vi "MCP23S17 Read LATCH.vi"(8 "error in (no error)":errorcluster, 10 "Addr":T1 items=["Addr-0"=0, "Addr-1"=4, "Addr-2"=2, "Addr-3"=6, "Addr-4"=1, "Addr-5"=5, "Addr-6"=3, "Addr-7"=7], 11 "handle":u32 format="%08x") -> (0 "error out":errorcluster, 2 "LATCH":u16, 3 "handle out":u32, 5 "buffer out B":string, 7 "buffer out A":string)   [LabVIEW 2018]
uses:
  PROJEKT/NIKO/Labview/Niko V4/FTDI SPI/Ctl/Sub Addr.ctl
  PROJEKT/NIKO/Labview/Niko V5/FTDI SPI/libMPSSE-SPI.lvlib
panel:
  out "string":string
  in  "Array U8":u8[](array[numeric])=[64, 18, 0, 128, 0, 0, 0, 0, 0, 0] format="%x"
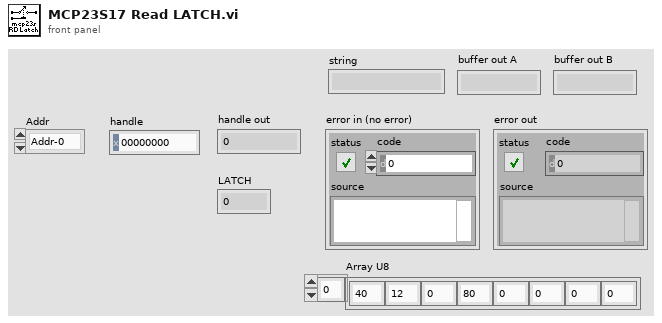
[diagram p1: front panel]
types:
  T1 = typedef "Sub Addr.ctl" = u16
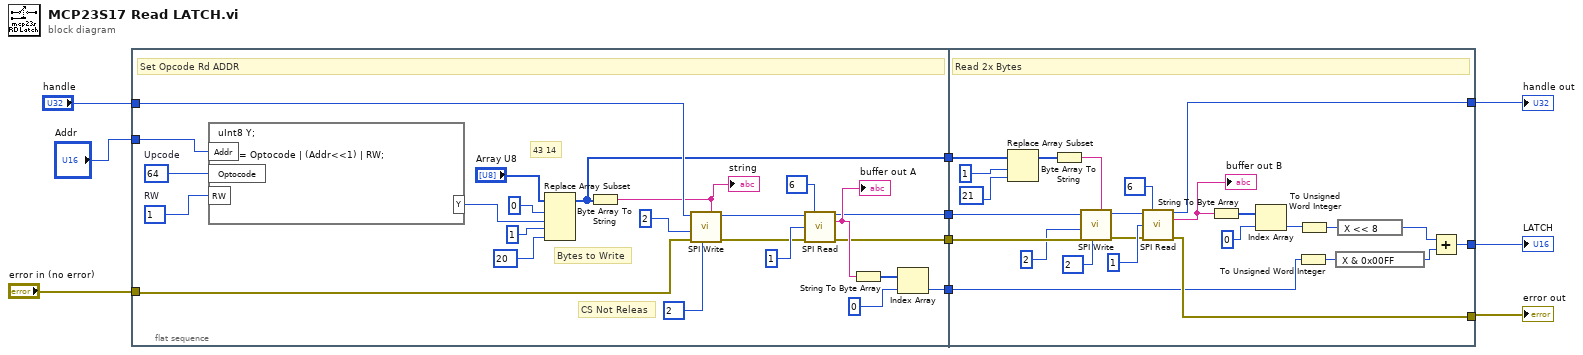
[diagram p0: block diagram]
diagram:
  n1 = flat-sequence {
    tunnel: "Addr" -> [w33]
    tunnel: "handle" -> [w29]
    tunnel: "error in (no error)" -> [w26]
    tunnel: [w14] -> w6
    tunnel: [w13] -> w5
    tunnel: [w12] -> w4
    tunnel: [w11] -> w3
    tunnel: [w57] -> w8
    tunnel: [w56] -> w2
    tunnel: [w51] -> w7
    tunnel: w6 -> [w50]
    tunnel: w5 -> [w46]
    tunnel: w4 -> [w44]
    tunnel: w3 -> [w35]
    frame #0 {
      w22 = u8 64  # Upcode
      w23 = u8 1  # RW
      # "CS Not Releas"
      # "Bytes to Write"
      # "43 14"
      # "Set Opcode Rd ADDR"
      n2 = formula code="uInt8 Y;\n      \n    Y = Optocode | (Addr<<1) | RW;"("Addr"=w33, "Optocode"=w22, "RW"=w23) -> ("Y"=w32:u8)
      n3 = Replace Array Subset(array="Array U8", new element #1=w32, index #1=0 ("index"), new element #2=u8 20, index #2=u8 1 ("new element/subarray")) -> (w14:u8[])
      n4 = Byte Array To String(unsigned byte array=w14) -> (string=w28:string)
      "string" <- w28
      n5 = call "SPI Write.vi"("buffer"=w28, "options"=u8 2, "error in (no error)"=w26, "Bytes To Send"=u32 2, "handle"=w29) -> ("error out"=w18:errorcluster, "handle out"=w19:u32)  [unwired: 4 in, 1 out]
      n6 = call "SPI Read.vi"("handle"=w19, "options"=u8 6, "sizeToTransfer"=u32 1, "error in (no error)"=w18) -> ("handle out"=w13:u32, "buffer out"=w15:string, "error out"=w12:errorcluster)  [unwired: 7 in, 2 out]
      "buffer out A" <- w15
      n7 = String To Byte Array(string=w15) -> (unsigned byte array=w16:u8[])
      n8 = Index Array(array=w16, index=0) -> (element=w11:u8)
    }
    frame #1 {
      # "Read 2x Bytes"
      n9 = Replace Array Subset(array=w50, new element=u8 21, index=u8 1 ("new element/subarray")) -> (w47:u8[])
      n10 = Byte Array To String(unsigned byte array=w47) -> (string=w45:string)
      n11 = call "SPI Write.vi"("buffer"=w45, "options"=u8 2, "error in (no error)"=w44, "Bytes To Send"=u32 2, "handle"=w46) -> ("error out"=w43:errorcluster, "handle out"=w42:u32)  [unwired: 4 in, 1 out]
      n12 = call "SPI Read.vi"("handle"=w42, "options"=u8 6, "sizeToTransfer"=u32 1, "error in (no error)"=w43) -> ("handle out"=w56:u32, "buffer out"=w55:string, "error out"=w57:errorcluster)  [unwired: 7 in, 2 out]
      "buffer out B" <- w55
      n13 = String To Byte Array(string=w55) -> (unsigned byte array=w54:u8[])
      n14 = Index Array(array=w54, index=0) -> (element=w52:u8)
      n15 = To Unsigned Word Integer(number=w35) -> (unsigned 16bit integer=w36:u16)
      n16 = To Unsigned Word Integer(number=w52) -> (unsigned 16bit integer=w39:u16)
      n17 = expression code="X & 0x00FF"(w36) -> (w37:u16)
      n18 = expression code="X << 8"(w39) -> (w38:u16)
      n19 = Add(x=w38, y=w37) -> (x+y=w51:u16)
    }
  }
  "error out" <- w8
  "handle out" <- w2
  "LATCH" <- w7
